vi "SplitWave.vi"(1 "Index":i32, 2 "SegmentPositions":u32[](array[numeric]), 3 "All Wave":T1 {"Phase (Pi)" min=-1.0 max=1.0 step=0.1 format="%.2f"; "Gap (us)" format="%.2f"; "Amplitude" format="%.2f"; "Duration (us)" format="%.2f"; "Frequency (MHz)" format="%.4f"}) -> (0 "Wave":T1 {"Phase (Pi)" min=-1.0 max=1.0 step=0.1 format="%.2f"; "Gap (us)" format="%.2f"; "Amplitude" format="%.2f"; "Duration (us)" format="%.2f"; "Frequency (MHz)" format="%.4f"})   [LabVIEW 2014]
uses:
  Wave.ctl
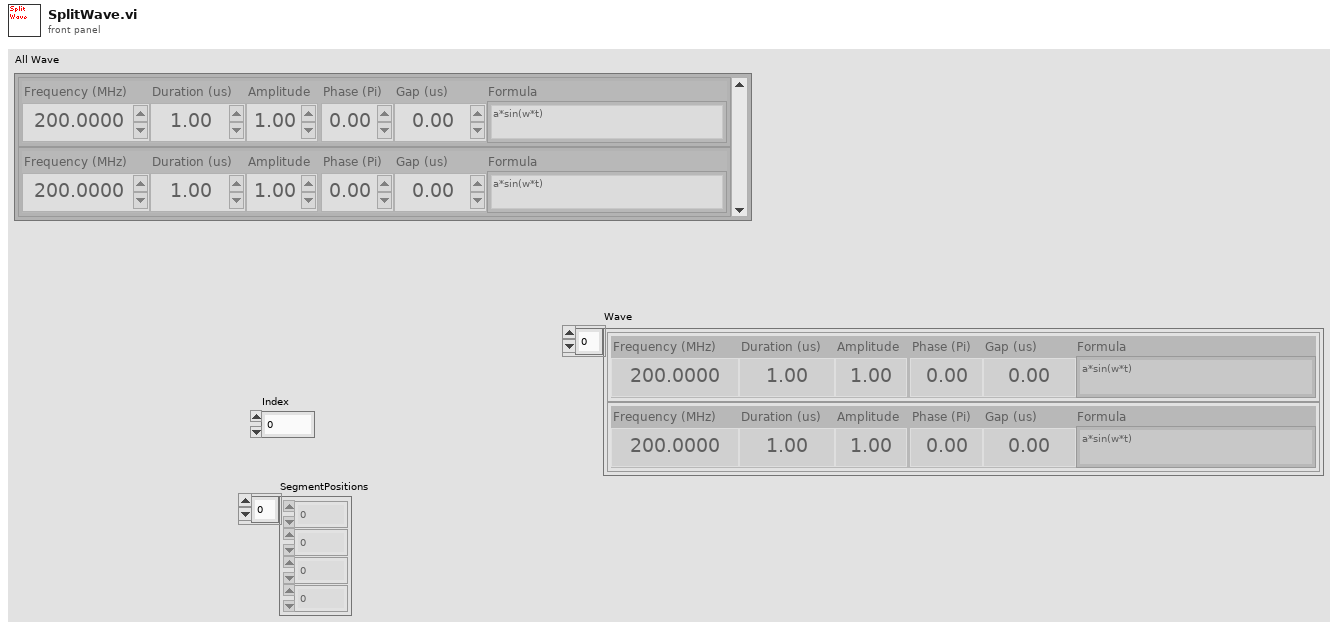
[diagram p1: front panel]
types:
  T1 = typedef "Wave.ctl" = cluster{"Frequency (MHz)":dbl, "Duration (us)":dbl, "Amplitude":dbl, "Phase (Pi)":dbl, "Gap (us)":dbl, "Formula":string}[]
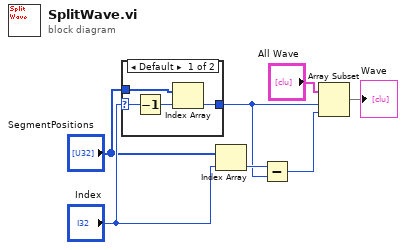
[diagram p0: block diagram]
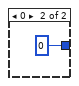
[diagram p2: hidden frame]
diagram:
  n1 = case shown="Default" "Index" {
    selector: "Index" -> [w11 _]
    tunnel: [w8 0] -> w6
    tunnel: "SegmentPositions" -> [w9 _]
    frame Default {
      n2 = Decrement(x=w11) -> (x-1=w10:i32)
      n3 = Index Array(array=w9, index=w10) -> (element=w8:u32)
    }
    frame 0 {
    }
  }
  n4 = Index Array(array="SegmentPositions", index="Index") -> (element=w7:u32)
  n5 = Subtract(x=w7, y=w6) -> (x-y=w5:u32)
  n6 = Array Subset(array="All Wave", index=w6, length=w5) -> (→"Wave":T1)
